vi "SENS_MULT_OUTP_DAT.vi"(0 "VISA IN":refnum<visa-resource-name>, 1 "ID":i32, 2 "Control Line Value":i32, 5 "error in":errorcluster, 7 "Channel":i32) -> (14 "VISA Out":refnum<visa-resource-name>, 19 "error out":errorcluster)   [LabVIEW 2018, in "PNA-X.lvlib"]
doc: "SENSe<cnum>:MULTiplexer<id>:OUTPut[:DATa] <num> \n1782\n\n(Read-Write) Sets or returns the control line value for the specified channel. \nParameters \n<cnum> Any existing channel number. If unspecified, value is set to 1. \n<id> Id of the external test set. If unspecified, Id is assumed to be 1. Must be \npreviously set by the SENSe:MULT:TYPE command. \n<numr> An integer specifying the decimal value of the control line. Values are obtained \nby adding weights from the following table that correspond to individual lines. \nHIGH =1; LOW=0. \nLine Weight \n1 1 \n2 2 \n3 4 \n4 8 \n5 16 \n6 32 \n7 64 \n8 128 \n0 - Sets all lines low \n255 - Sets all lines high \nExamples SENS3:MULT1:OUTP 48 'For test set 1 on channel 3, sets lines 5 \nand 6 to HIGH state; all other lines are set to LOW state. \nQuery Syntax SENSe<cnum>:MULTiplexer<id>:OUTPut[:DATa]? \nReturn Type Numeric \nDefault Not Applicable \nSENSe:MULTiplexer<id>:PORT<pnum>CATalog? \n1783\n\n(Read-Only) Returns a comma-separated list of valid port selections for the specified port. \nParameters \n<id> Id of the external test set. If unspecified, Id is assumed to be 1. Must be \npreviously set by the SENSe:MULT:TYPE command. \n<pnum> Integer - Input port number for which to return valid Output port selections. \nRead the number of input ports for the test set using SENS:MULT:INCount? \nExamples SENS:MULT1:PORT3:CAT? ' returns the valid port selections for \nport 3 \nReturn Type String \nDefault Not Applicable"
uses:
  PNA-X.lvlib
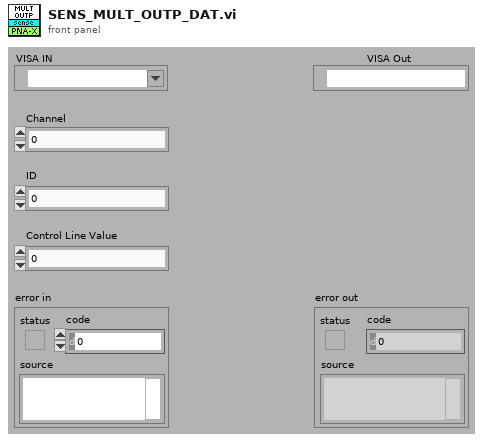
[diagram p1: front panel]
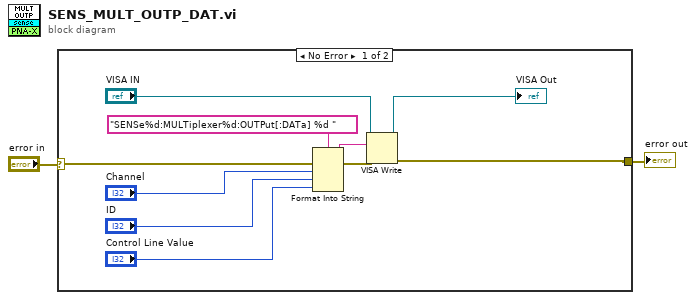
[diagram p0: block diagram]
diagram:
  n1 = case shown="No Error" "error in" {
    selector: "error in" -> [w12 w13]
    tunnel: [w7 w13] -> w1
    frame No Error {
      n2 = Format Into String(format string="SENSe%d:MULTiplexer%d:OUTPut[:DATa] %d " ("Cmdline"), error in=w12, "Channel", "ID", "Control Line Value") -> (resulting string=w10:string, error out=w11:errorcluster)  [unwired: 1 in]
      n3 = VISA Write(VISA resource name="VISA IN", write buffer=w10, error in (no error)=w11) -> (VISA resource name out=→"VISA Out":refnum<visa-resource-name>, error out=w7:errorcluster)  [unwired: 1 out]
    }
    frame Error {
    }
  }
  "error out" <- w1
